vi "Process Data In 2 Byte Chunks.vi"(10 "DATA IN":u8[](array[numeric])) -> (2 "Data Out":u16[](array[numeric]) format="%x")   [LabVIEW 2020]
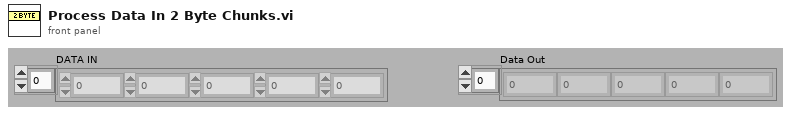
[diagram p1: front panel]
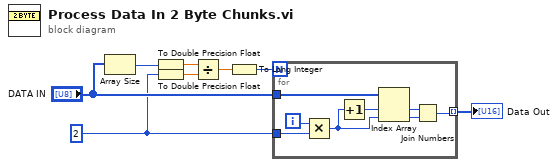
[diagram p0: block diagram]
diagram:
  w2 = 2 ("Chunk Size")
  n1 = Array Size(array="DATA IN") -> (size(s)=w7:i32)
  n2 = To Double Precision Float(number=w7) -> (double precision float=w5:dbl)
  n3 = To Double Precision Float(number=w2) -> (double precision float=w4:dbl)
  n4 = Divide(x=w5, y=w4) -> (x/y=w6:dbl)
  n5 = To Long Integer(number=w6) -> (32bit integer=w3:i32)
  n6 = for {
    N: w3 -> [_]
    tunnel: "DATA IN" -> [w16]
    tunnel: [w10] -> w1 mode=indexing
    tunnel: w2 -> [w9]
    i -> [w14]
    n7 = Multiply(x=w14, y=w9) -> (x*y=w13:i32)
    n8 = Increment(x=w13) -> (x+1=w15:i32)
    n9 = Index Array(array=w16, index #1=w15, index #2=w13) -> (element #1=w12:u8, element #2=w11:u8)
    n10 = Join Numbers(hi=w12, lo=w11) -> ((hi.lo)=w10:u16)
  }
  "Data Out" <- w1
